vi "OptPumpLeakage.vi"() -> ()   [LabVIEW 2012]
panel:
  in  "How Often Recool?":i32
  out "Bright Counts":i32
  in  "Bright Threshold":dbl
  out "Leakage\nFluorescence":dbl
  in  "stop":bool
  in  "How many runs?":i32
  out "Red Off Pockel On":dbl
  out "Pockel On":dbl
  in  "PMT Sample Time (secs)":dbl=0.05 format="%0.2f"
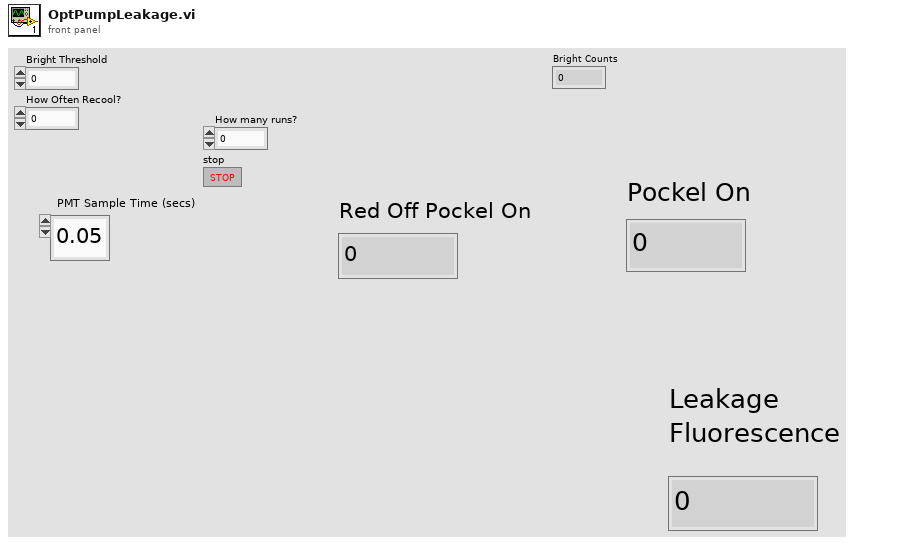
[diagram p1: front panel]
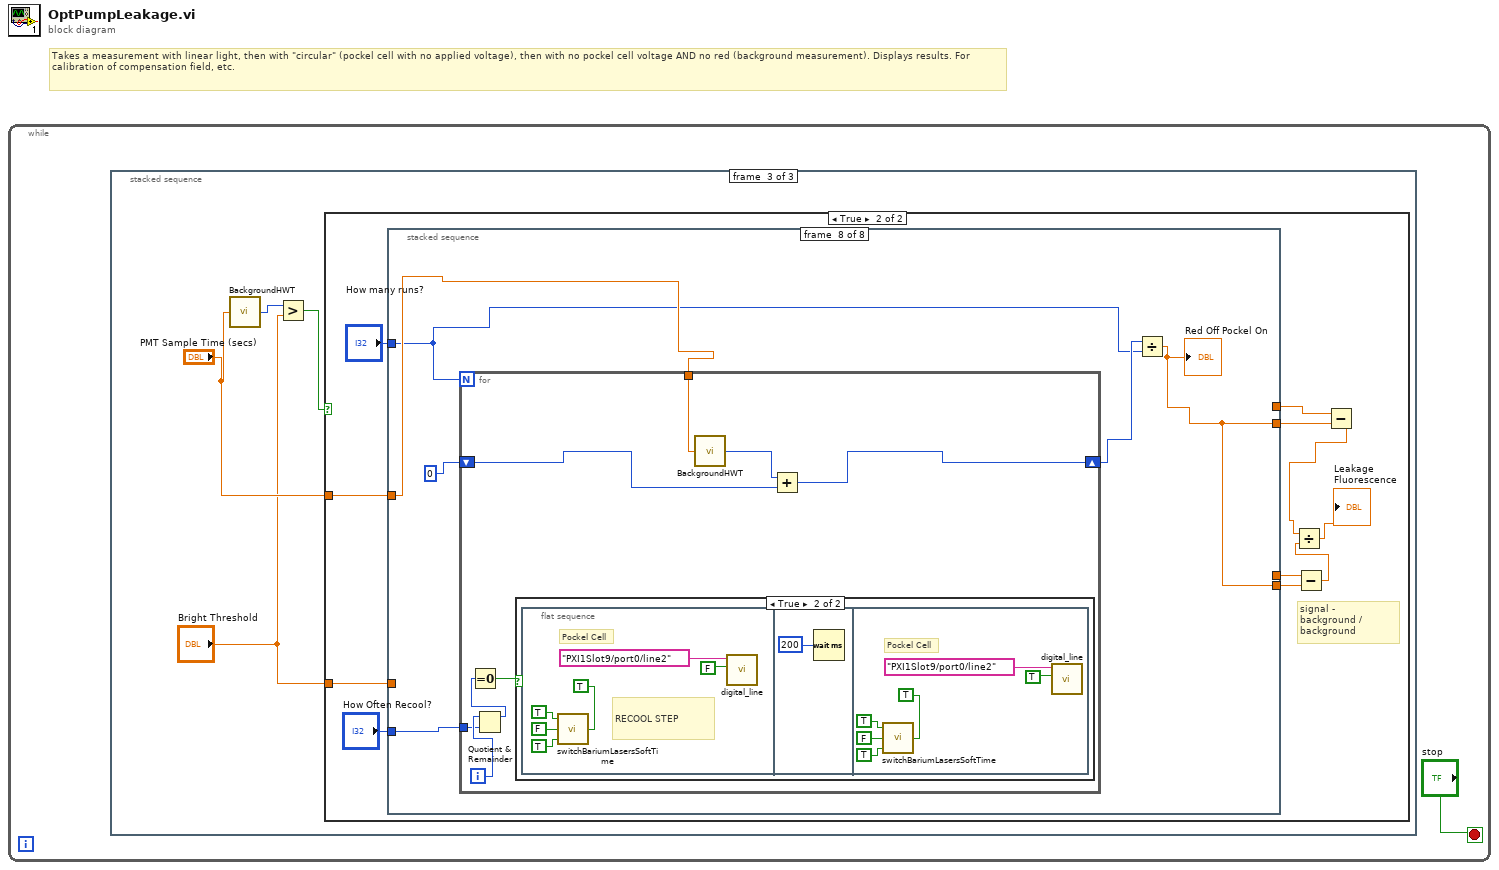
[diagram p0: block diagram]
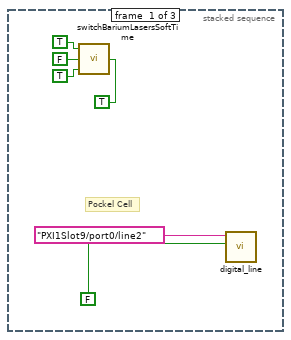
[diagram p2: hidden frame]
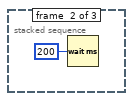
[diagram p3: hidden frame]
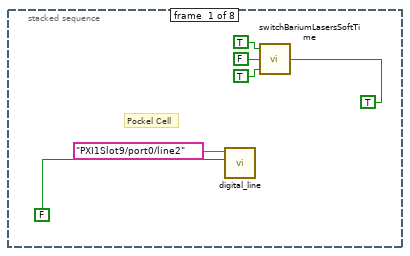
[diagram p5: hidden frame]
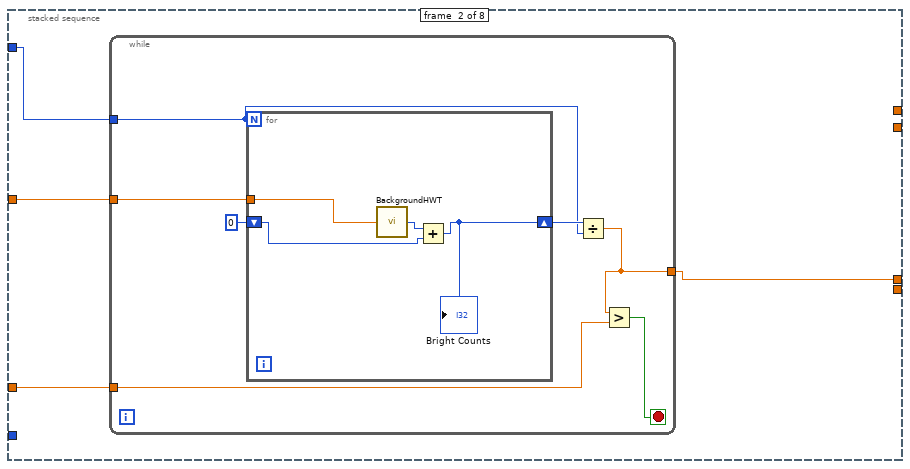
[diagram p6: hidden frame]
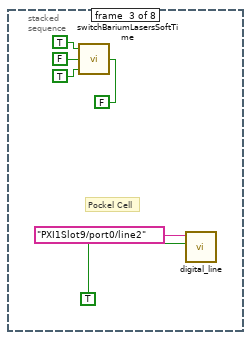
[diagram p7: hidden frame]
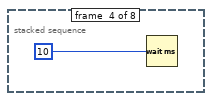
[diagram p8: hidden frame]
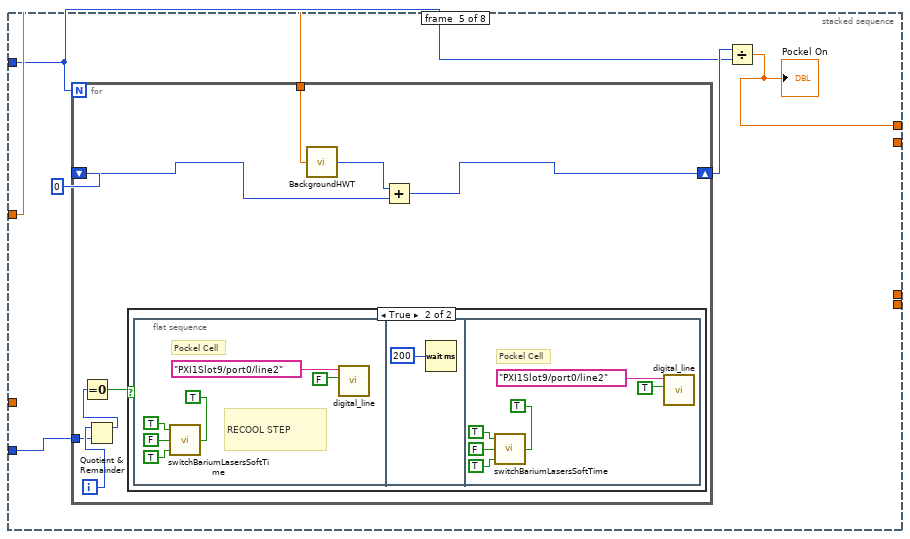
[diagram p9: hidden frame]
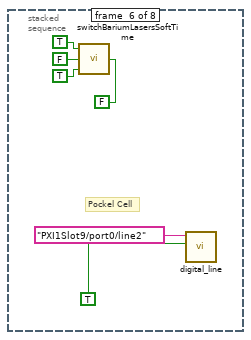
[diagram p11: hidden frame]
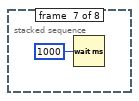
[diagram p12: hidden frame]
diagram:
  # "Takes a measurement with linear light, then with \"circular\" (pockel cell with no applied voltage), then with no pockel cell voltage AND no red (background measurement). Displays results. For calibration of compensation field, etc."
  n1 = while {
    stop <- "stop" stop-if-true
    n2 = stacked-sequence {
      frame #0 {
        # "Pockel Cell"
        n3 = call "switchBariumLasersSoftTime.vi"("650"=TRUE, "614"=TRUE, "1762"=FALSE, "493"=TRUE) -> ()  [unwired: 2 in]
        n4 = call "digital_line.vi"("Boolean"=FALSE ("Pockel"), "lines"=tag "PXI1Slot9/port0/line2") -> ()  [unwired: 5 in, 1 out]
      }
      frame #1 {
        n5 = Wait (ms)(milliseconds to wait=u32 200) -> ()  [unwired: 1 out]
      }
      frame #2 {
        n6 = call "BackgroundHWT.vi"("Sample Time(seconds)"="PMT Sample Time (secs)") -> ("Counts"=w11:i32)
        n7 = Greater?(x=w11, y="Bright Threshold") -> (0:w9:bool)
        n8 = case shown="True" w9 {
          tunnel: "PMT Sample Time (secs)" -> [_ w17]
          tunnel: "Bright Threshold" -> [_ w14]
          frame False {
          }
          frame True {
            # "signal - background / background"
            n9 = stacked-sequence {
              tunnel: [_ _ _ _ w55 _ _ _] -> w23
              tunnel: [_ _ _ _ _ _ _ w91] -> w22
              tunnel: "How many runs?" -> [_ w32 _ _ w53 _ _ w87]
              tunnel: w17 -> [_ w33 _ _ w54 _ _ w90]
              tunnel: [_ _ _ _ _ _ _ w91] -> w16
              tunnel: [_ w31 _ _ _ _ _ _] -> w15
              tunnel: w14 -> [_ w30 _ _ _ _ _ _]
              tunnel: "How Often Recool?" -> [_ _ _ _ w52 _ _ w89]
              frame #0 {
                # "Pockel Cell"
                n10 = call "digital_line.vi"("Boolean"=FALSE ("Pockel"), "lines"=tag "PXI1Slot9/port0/line2") -> ()  [unwired: 5 in, 1 out]
                n11 = call "switchBariumLasersSoftTime.vi"("650"=TRUE, "614"=TRUE, "1762"=FALSE, "493"=TRUE) -> ()  [unwired: 2 in]
              }
              frame #1 {
                n12 = while {
                  tunnel: [w36] -> w31
                  tunnel: w33 -> [w39]
                  tunnel: w32 -> [w35]
                  tunnel: w30 -> [w34]
                  stop <- w40 stop-if-true
                  n13 = for {
                    N: w35 -> [_]
                    tunnel: w39 -> [w44]
                    shift-right: [w41] -> w37
                    shift-left: 0 ("Counts") -> [w42]
                    n14 = call "BackgroundHWT.vi"("Sample Time(seconds)"=w44) -> ("Counts"=w43:i32)
                    n15 = Add(x=w43, y=w42) -> (x+y=w41:i32)
                    "Bright Counts" <- w41
                  }
                  n16 = Divide(x=w37, y=w35) -> (x/y=w36:dbl)
                  n17 = Greater?(x=w36, y=w34) -> (0:w40:bool)
                }
              }
              frame #2 {
                # "Pockel Cell"
                n18 = call "switchBariumLasersSoftTime.vi"("650"=FALSE, "614"=TRUE, "1762"=FALSE, "493"=TRUE) -> ()  [unwired: 2 in]
                n19 = call "digital_line.vi"("Boolean"=TRUE ("Pockel"), "lines"=tag "PXI1Slot9/port0/line2") -> ()  [unwired: 5 in, 1 out]
              }
              frame #3 {
                n20 = Wait (ms)(milliseconds to wait=u32 10) -> ()  [unwired: 1 out]
              }
              frame #4 {
                n21 = for {
                  N: w53 -> [_]
                  tunnel: w54 -> [w65]
                  shift-right: [w63] -> w56
                  shift-left: 0 -> [w64]
                  tunnel: w52 -> [w60]
                  i -> [w61]
                  n22 = Quotient & Remainder(x=w61, y=w60) -> (x-y*floor(x/y)=w59:i32)  [unwired: 1 out]
                  n23 = Equal To 0?(x=w59) -> (x = 0?=w58:bool)
                  n24 = case shown="True" w58 {
                    frame False {
                    }
                    frame True {
                      n25 = flat-sequence {
                        frame #0 {
                          # "RECOOL STEP"
                          # "Pockel Cell"
                          n26 = call "switchBariumLasersSoftTime.vi"("650"=TRUE, "614"=TRUE, "1762"=FALSE, "493"=TRUE) -> ()  [unwired: 2 in]
                          n27 = call "digital_line.vi"("Boolean"=FALSE ("Pockel"), "lines"=tag "PXI1Slot9/port0/line2") -> ()  [unwired: 5 in, 1 out]
                        }
                        frame #1 {
                          n28 = Wait (ms)(milliseconds to wait=u32 200) -> ()  [unwired: 1 out]
                        }
                        frame #2 {
                          # "Pockel Cell"
                          n29 = call "switchBariumLasersSoftTime.vi"("650"=TRUE, "614"=TRUE, "1762"=FALSE, "493"=TRUE) -> ()  [unwired: 2 in]
                          n30 = call "digital_line.vi"("Boolean"=TRUE ("Pockel"), "lines"=tag "PXI1Slot9/port0/line2") -> ()  [unwired: 5 in, 1 out]
                        }
                      }
                    }
                  }
                  n31 = call "BackgroundHWT.vi"("Sample Time(seconds)"=w65) -> ("Counts"=w62:i32)
                  n32 = Add(x=w62, y=w64) -> (x+y=w63:i32)
                }
                n33 = Divide(x=w56, y=w53) -> (x/y=w55:dbl)
                "Pockel On" <- w55
              }
              frame #5 {
                # "Pockel Cell"
                n34 = call "switchBariumLasersSoftTime.vi"("650"=FALSE, "614"=TRUE, "1762"=FALSE, "493"=TRUE) -> ()  [unwired: 2 in]
                n35 = call "digital_line.vi"("Boolean"=TRUE ("Pockel"), "lines"=tag "PXI1Slot9/port0/line2") -> ()  [unwired: 5 in, 1 out]
              }
              frame #6 {
                n36 = Wait (ms)(milliseconds to wait=u32 1000) -> ()  [unwired: 1 out]
              }
              frame #7 {
                n37 = for {
                  N: w87 -> [_]
                  tunnel: w90 -> [w99]
                  shift-right: [w97] -> w88
                  shift-left: 0 -> [w98]
                  tunnel: w89 -> [w92]
                  i -> [w95]
                  n38 = Quotient & Remainder(x=w95, y=w92) -> (x-y*floor(x/y)=w94:i32)  [unwired: 1 out]
                  n39 = Equal To 0?(x=w94) -> (x = 0?=w93:bool)
                  n40 = case shown="True" w93 {
                    frame False {
                    }
                    frame True {
                      n41 = flat-sequence {
                        frame #0 {
                          # "RECOOL STEP"
                          # "Pockel Cell"
                          n42 = call "switchBariumLasersSoftTime.vi"("650"=TRUE, "614"=TRUE, "1762"=FALSE, "493"=TRUE) -> ()  [unwired: 2 in]
                          n43 = call "digital_line.vi"("Boolean"=FALSE ("Pockel"), "lines"=tag "PXI1Slot9/port0/line2") -> ()  [unwired: 5 in, 1 out]
                        }
                        frame #1 {
                          n44 = Wait (ms)(milliseconds to wait=u32 200) -> ()  [unwired: 1 out]
                        }
                        frame #2 {
                          # "Pockel Cell"
                          n45 = call "switchBariumLasersSoftTime.vi"("650"=TRUE, "614"=TRUE, "1762"=FALSE, "493"=TRUE) -> ()  [unwired: 2 in]
                          n46 = call "digital_line.vi"("Boolean"=TRUE ("Pockel"), "lines"=tag "PXI1Slot9/port0/line2") -> ()  [unwired: 5 in, 1 out]
                        }
                      }
                    }
                  }
                  n47 = call "BackgroundHWT.vi"("Sample Time(seconds)"=w99) -> ("Counts"=w96:i32)
                  n48 = Add(x=w96, y=w98) -> (x+y=w97:i32)
                }
                n49 = Divide(x=w88, y=w87) -> (x/y=w91:dbl)
                "Red Off Pockel On" <- w91
              }
            }
            n50 = Subtract(x=w15, y=w16) -> (x-y=w20:dbl)
            n51 = Subtract(x=w23, y=w22) -> (x-y=w21:dbl)
            n52 = Divide(x=w21, y=w20) -> (x/y=→"Leakage\nFluorescence":dbl)
          }
        }
      }
    }
  }
